vi "温度湿度监测界面.vi"() -> ()   [LabVIEW 2016, in "环境动力监测库.lvlib"]
uses:
  <vilib>/Utility/config.llb/NI_LVConfig.lvlib
  <vilib>/ptbypt/NI_PtbyPt.lvlib
panel:
  in  "解除告警":bool
  out "告警内容":string
  in  "高温告警启用":bool
  out "湿度显示":dbl=21.0 format="%.2f %%"
  out "湿度":dbl(graph)
  out "温度显示":dbl=21.0 format="%.2f ℃"
  out "温度":dbl(graph)
  in  "湿度下限告警点":dbl
  in  "湿度上限告警点":dbl
  in  "室温下限告警点":dbl
  in  "室温上限告警点":dbl
  # "℃"
  # "℃"
  # "%"
  # "%"
  # "温湿度监测"
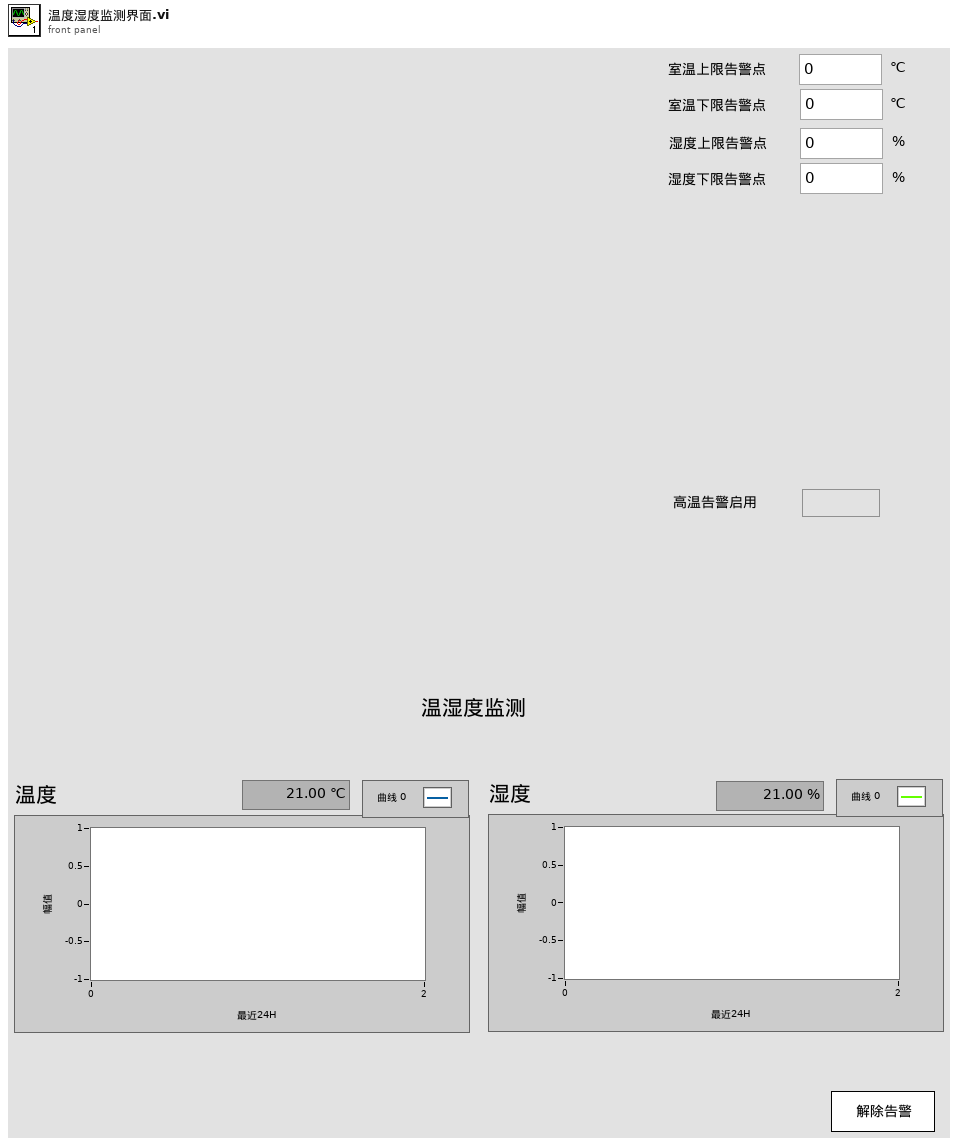
[diagram p1: front panel]
types:
  T1 = enum16{"报警状态监测", "报警确认", "仪器断电", "市电断电", "工控机关机", "取消告警", "结束"}
  T2 = typedef "NI_LVConfig.lvlib/Config Data RefNum.ctl" = refnum<k1>
  T3 = cluster{"漏水监测配置":cluster{"监测项描述:输出":string, "端口:":enum16{"AI0", "AI1", "AI2", "AI3", "AI4", "DI0", "DI1", "DI2", "DI3", "DI4", "DO0", "DO1", "DO2", "DO3", "DO4", "X0", "X1", "X2", "X3", "X4", "X5", "X6", "X7", "X8", "X9"}, "告警参数:":enum32{"禁用告警", "闭合告警", "断开告警"}, "传感器型号:":enum16{"PLC", "ZLAN"}, "声光告警启用":bool}, "门禁开关监测配置":cluster{"监测项描述:输出":string, "端口:":enum16{"AI0", "AI1", "AI2", "AI3", "AI4", "DI0", "DI1", "DI2", "DI3", "DI4", "DO0", "DO1", "DO2", "DO3", "DO4", "X0", "X1", "X2", "X3", "X4", "X5", "X6", "X7", "X8", "X9"}, "告警参数:":enum32{"禁用告警", "闭合告警", "断开告警"}, "传感器型号:":enum16{"PLC", "ZLAN"}, "声光告警启用":bool}, "门禁开关监测配置2":cluster{"监测项描述:输出":string, "端口:":enum16{"AI0", "AI1", "AI2", "AI3", "AI4", "DI0", "DI1", "DI2", "DI3", "DI4", "DO0", "DO1", "DO2", "DO3", "DO4", "X0", "X1", "X2", "X3", "X4", "X5", "X6", "X7", "X8", "X9"}, "告警参数:":enum32{"禁用告警", "闭合告警", "断开告警"}, "传感器型号:":enum16{"PLC", "ZLAN"}, "声光告警启用":bool}, "温湿度监测配置":cluster{"监测项描述:输出":string, "端口:":enum16{"AI0", "AI1", "AI2", "AI3", "AI4", "DI0", "DI1", "DI2", "DI3", "DI4", "DO0", "DO1", "DO2", "DO3", "DO4", "X0", "X1", "X2", "X3", "X4", "X5", "X6", "X7", "X8", "X9"}, "告警参数:":enum32{"禁用告警", "闭合告警", "断开告警"}, "传感器型号:":enum16{"PLC", "ZLAN"}, "声光告警启用":bool}, "烟雾监测配置":cluster{"监测项描述:输出":string, "端口:":enum16{"AI0", "AI1", "AI2", "AI3", "AI4", "DI0", "DI1", "DI2", "DI3", "DI4", "DO0", "DO1", "DO2", "DO3", "DO4", "X0", "X1", "X2", "X3", "X4", "X5", "X6", "X7", "X8", "X9"}, "告警参数:":enum32{"禁用告警", "闭合告警", "断开告警"}, "传感器型号:":enum16{"PLC", "ZLAN"}, "声光告警启用":bool}, "冰箱监测配置":cluster{"监测项描述:输出":string, "端口:":enum16{"AI0", "AI1", "AI2", "AI3", "AI4", "DI0", "DI1", "DI2", "DI3", "DI4", "DO0", "DO1", "DO2", "DO3", "DO4", "X0", "X1", "X2", "X3", "X4", "X5", "X6", "X7", "X8", "X9"}, "告警参数:":enum32{"禁用告警", "闭合告警", "断开告警"}, "传感器型号:":enum16{"PLC", "ZLAN"}, "声光告警启用":bool}, "排气扇监测配置":cluster{"监测项描述:输出":string, "端口:":enum16{"AI0", "AI1", "AI2", "AI3", "AI4", "DI0", "DI1", "DI2", "DI3", "DI4", "DO0", "DO1", "DO2", "DO3", "DO4", "X0", "X1", "X2", "X3", "X4", "X5", "X6", "X7", "X8", "X9"}, "告警参数:":enum32{"禁用告警", "闭合告警", "断开告警"}, "传感器型号:":enum16{"PLC", "ZLAN"}, "声光告警启用":bool}, "红外入侵监测配置":cluster{"监测项描述:输出":string, "端口:":enum16{"AI0", "AI1", "AI2", "AI3", "AI4", "DI0", "DI1", "DI2", "DI3", "DI4", "DO0", "DO1", "DO2", "DO3", "DO4", "X0", "X1", "X2", "X3", "X4", "X5", "X6", "X7", "X8", "X9"}, "告警参数:":enum32{"禁用告警", "闭合告警", "断开告警"}, "传感器型号:":enum16{"PLC", "ZLAN"}, "声光告警启用":bool}, "振动监测配置":cluster{"监测项描述:输出":string, "端口:":enum16{"AI0", "AI1", "AI2", "AI3", "AI4", "DI0", "DI1", "DI2", "DI3", "DI4", "DO0", "DO1", "DO2", "DO3", "DO4", "X0", "X1", "X2", "X3", "X4", "X5", "X6", "X7", "X8", "X9"}, "告警参数:":enum32{"禁用告警", "闭合告警", "断开告警"}, "传感器型号:":enum16{"PLC", "ZLAN"}, "声光告警启用":bool}}
  T4 = cluster{"监测项描述:输出":string, "端口:":enum16{"AI0", "AI1", "AI2", "AI3", "AI4", "DI0", "DI1", "DI2", "DI3", "DI4", "DO0", "DO1", "DO2", "DO3", "DO4", "X0", "X1", "X2", "X3", "X4", "X5", "X6", "X7", "X8", "X9"}, "告警参数:":enum32{"禁用告警", "闭合告警", "断开告警"}, "传感器型号:":enum16{"PLC", "ZLAN"}, "声光告警启用":bool}
  T5 = enum16{"AI0", "AI1", "AI2", "AI3", "AI4", "DI0", "DI1", "DI2", "DI3", "DI4", "DO0", "DO1", "DO2", "DO3", "DO4", "X0", "X1", "X2", "X3", "X4", "X5", "X6", "X7", "X8", "X9"}
  T6 = cluster{"状态":cluster{"R0":i16, "R1":i16, "R2":i16, "R3":i16, "R4":i16, "R5":i16, "R6":i16, "R7":i16, "R8":i16, "R9":i16, "R10":i16, "R11":i16, "R12":i16, "R13":i16, "R14":i16, "R15":i16, "R16":i16, "R17":i16, "R18":i16, "R19":i16, "R20":i16, "R21":i16, "R22":i16, "R23":i16, "R24":i16, "R25":i16, "R26":i16, "R27":i16, "R28":i16, "R29":i16, "R30":i16, "R31":i16, "R32":i16, "R33":i16, "R34":i16, "R35":i16, "R36":i16, "R37":i16, "R38":i16, "R39":i16}, "输入状态":bool[], "输出状态":bool[], "参数设置":cluster{"R100":i16, "R101":i16, "R102":i16, "R103":i16, "R104":i16, "R105":i16, "R106":i16, "R107":i16, "R108":i16, "R109":i16, "R110":i16, "R111":i16, "R112":i16, "R113":i16, "R114":i16, "R115":i16, "R116":i16, "R117":i16, "R118":i16, "R119":i16, "R120":i16, "R121":i16, "R122":i16, "R123":i16}, "转换值":cluster{"AD0":sgl, "AD1":sgl, "AD2":sgl, "AD3":sgl, "AD4":sgl, "AD5":sgl}}
  T7 = cluster{"状态":cluster{"R0":i16, "R1":i16, "R2":i16, "R3":i16, "R4":i16, "R5":i16, "R6":i16, "R7":i16, "R8":i16, "R9":i16, "R10":i16, "R11":i16, "R12":i16, "R13":i16, "R14":i16, "R15":i16, "R16":i16, "R17":i16, "R18":i16, "R19":i16, "R20":i16, "R21":i16, "R22":i16, "R23":i16, "R24":i16, "R25":i16, "R26":i16, "R27":i16, "R28":i16, "R29":i16, "R30":i16, "R31":i16, "R32":i16, "R33":i16, "R34":i16, "R35":i16, "R36":i16, "R37":i16, "R38":i16, "R39":i16, "R40":i16, "R41":i16, "R42":i16, "R43":i16, "R44":i16, "R45":i16, "R46":i16, "R47":i16, "R48":i16, "R49":i16, "R50":i16, "R51":i16, "R52":i16, "R53":i16, "R54":i16, "R55":i16, "R56":i16, "R57":i16, "R58":i16, "R59":i16, "R60":i16, "R61":i16, "R62":i16, "R63":i16, "R64":i16, "R65":i16, "R66":i16, "R67":i16, "R68":i16, "R69":i16}, "输入状态":bool[], "输出状态":bool[], "报警簇":bool[], "参数设置":cluster{"R100":i16, "R101":i16, "R102":i16, "R103":i16, "R104":i16, "R105":i16, "R106":i16, "R107":i16, "R108":i16, "R109":i16, "R110":i16, "R111":i16, "R112":i16, "R113":i16, "R114":i16, "R115":i16, "R116":i16, "R117":i16, "R118":i16, "R119":i16, "R120":i16, "R121":i16, "R122":i16, "R123":i16, "R124":i16}, "转换值":cluster{"AD0":sgl, "AD1":sgl, "AD2":sgl, "AD3":sgl, "AD4":sgl, "AD5":sgl}, "看门狗启用":bool, "氨氮模块名称":string, "总磷模块名称":string}
  T8 = cluster{"AD0":dbl, "AD1":dbl, "AD2":dbl, "AD3":dbl, "AD4":dbl, "AD5":dbl, "AD6":dbl, "AD7":dbl}
  T9 = cluster{"命令":string, cluster{"starting address":u16, "holding register value":u16}}
  T10 = cluster{"温湿度":cluster{"状态":bool, "温度:":sgl, "湿度:":sgl, "详情  ":bool}, "空调":cluster{"状态":bool, "机柜温度:":sgl, "压缩机:":enum16{"停止", "运行"}, "电加热:":enum16{"停止", "运行"}, "详情  ":bool}, "排气扇":cluster{"排气扇:":enum16{"关闭", "打开"}, "详情  ":bool}, "冰箱":cluster{"冰箱:":enum16{"关闭", "打开"}, "详情  ":bool}}
  T11 = cluster{"漏水监测输出":cluster{"漏水监测告警":bool, "告警内容":string}, "门禁监测输出":cluster{"门禁监测告警":bool, "告警内容":string}, "门禁监测输出2":cluster{"门禁监测告警":bool, "告警内容":string}, "温湿度监测输出":cluster{"温湿度监测告警":bool, "告警内容":string}, "烟雾监测输出":cluster{"烟雾监测告警":bool, "告警内容":string}, "空调监测输出":cluster{"空调监测告警":bool, "告警内容":string}, "自动重合闸输出":cluster{"自动重合闸告警":bool, "告警内容":string}, "红外入侵输出":cluster{"红外入侵告警":bool, "告警内容":string}, "振动输出":cluster{"振动告警":bool, "告警内容":string}, "UPS输出":cluster{"UPS告警":bool, "告警内容":string}, "蓄电池输出":cluster{"蓄电池告警":bool, "告警内容":string}, "蓄电池输出2":cluster{"蓄电池告警":bool, "告警内容":string}, "GPS输出":cluster{"定位告警":bool, "告警内容":string}, "北斗输出":cluster{"定位告警":bool, "告警内容":string}, "气象输出":cluster{"气象告警":bool, "告警内容":string}}
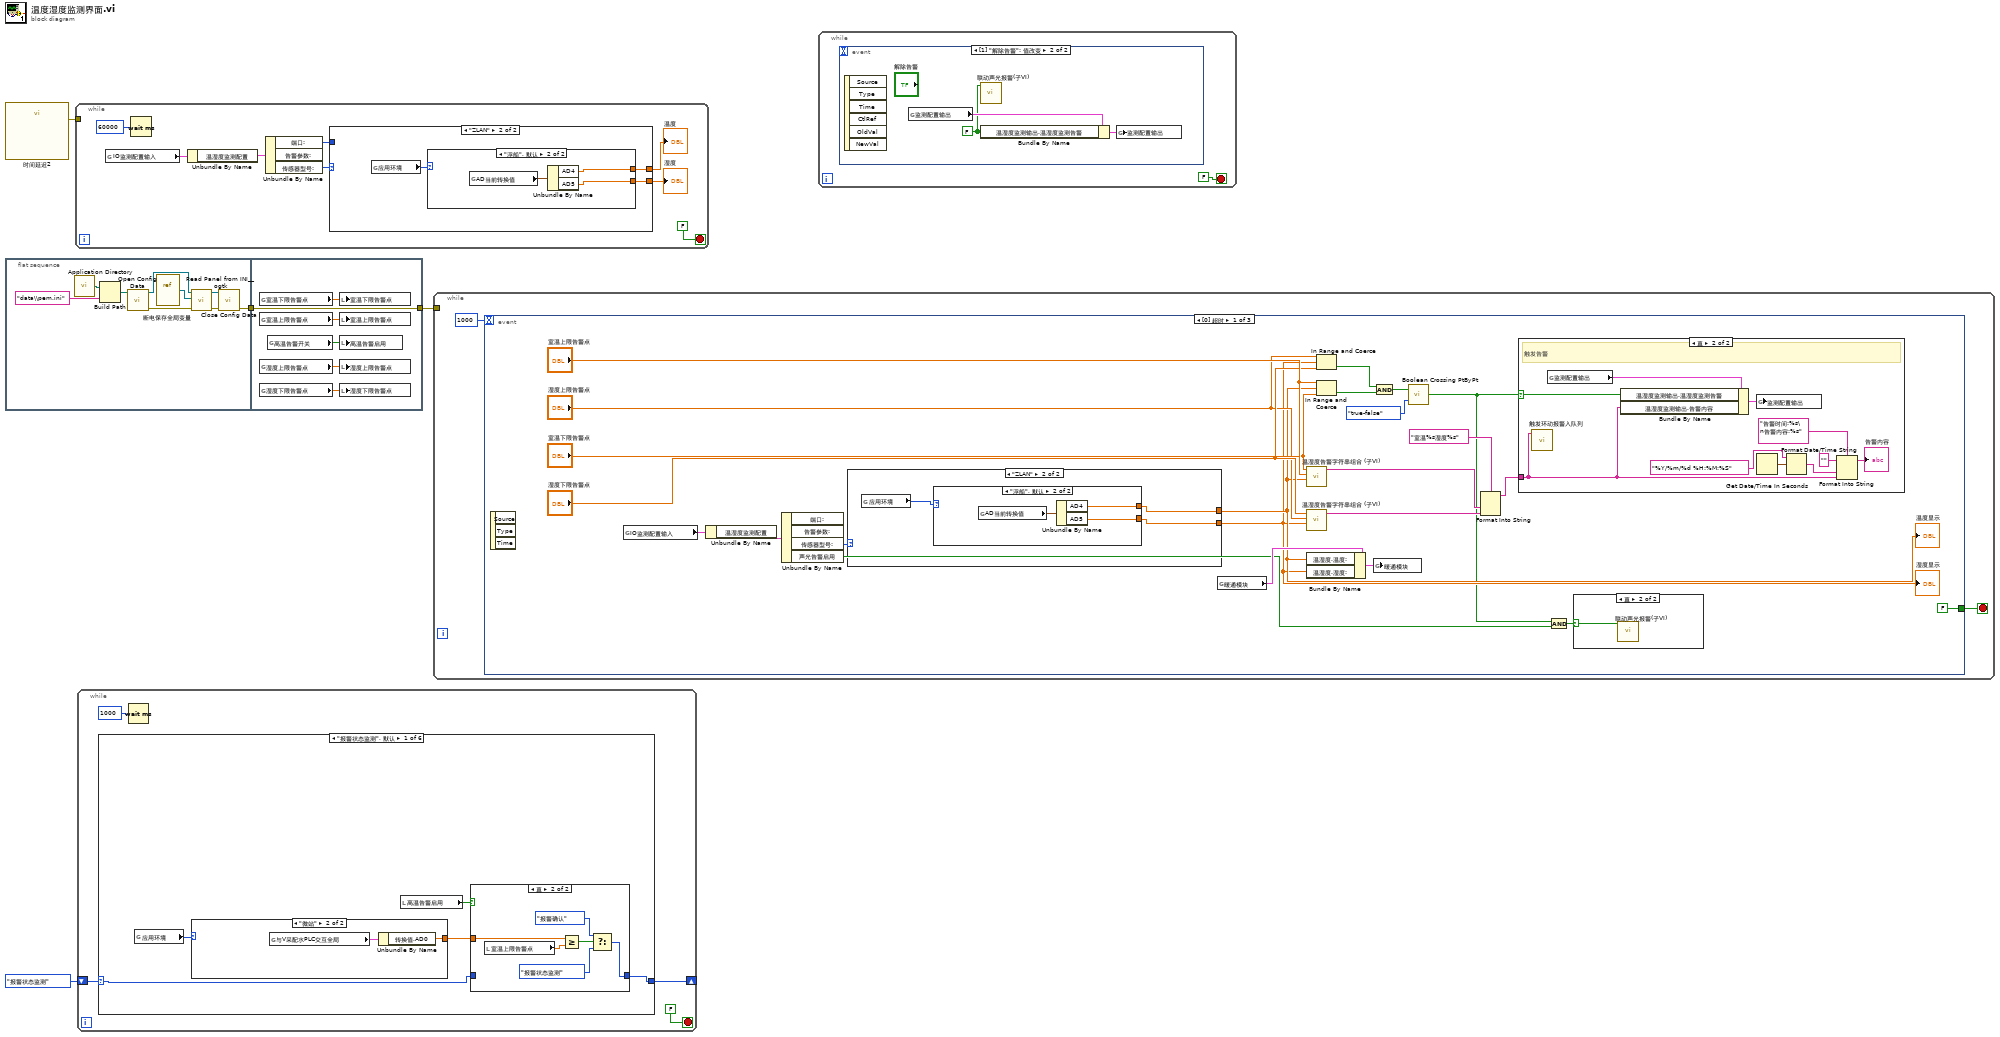
[diagram p0: block diagram]
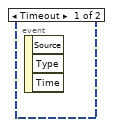
[diagram p2: hidden frame]
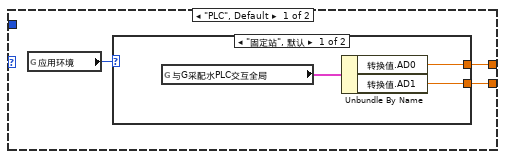
[diagram p3: hidden frame]
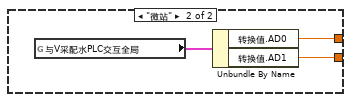
[diagram p4: hidden frame]
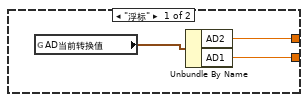
[diagram p5: hidden frame]
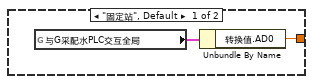
[diagram p6: hidden frame]
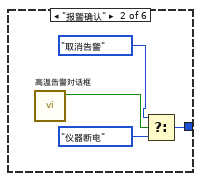
[diagram p8: hidden frame]
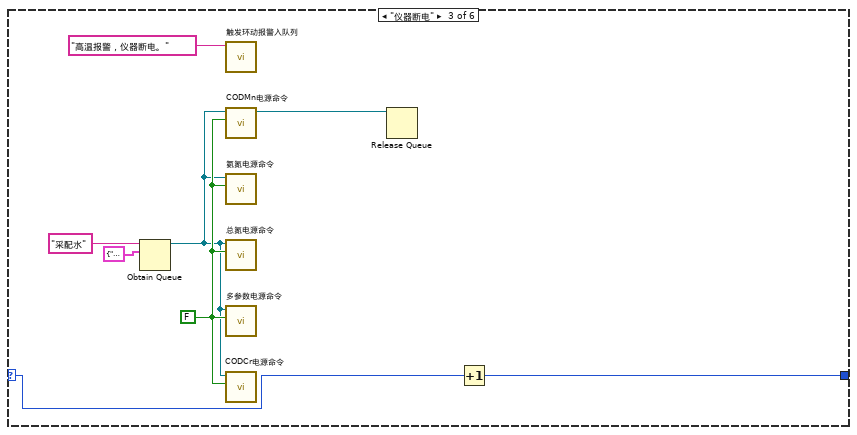
[diagram p9: hidden frame]
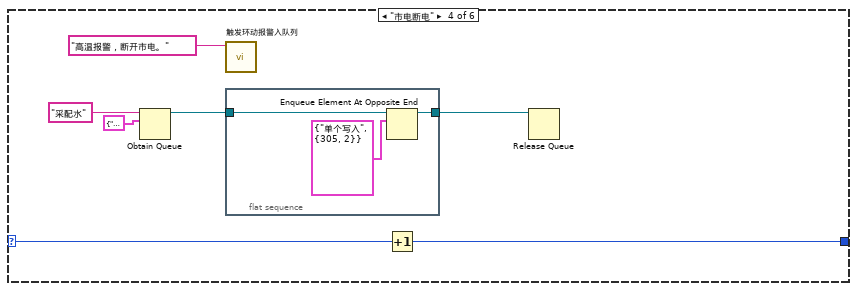
[diagram p10: hidden frame]
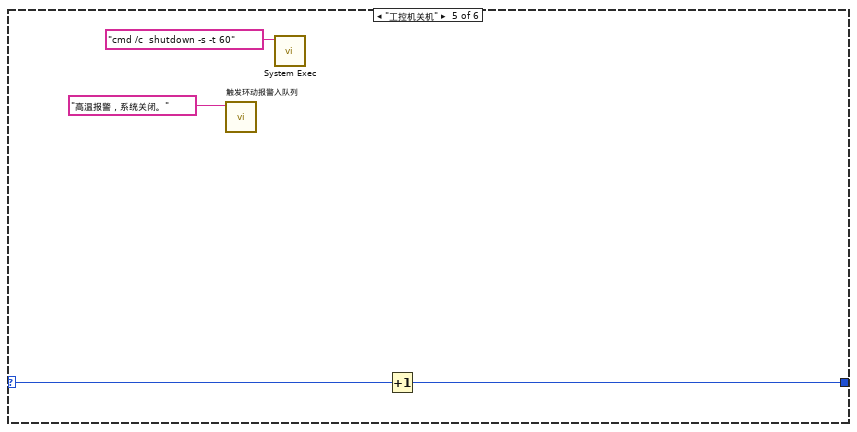
[diagram p11: hidden frame]
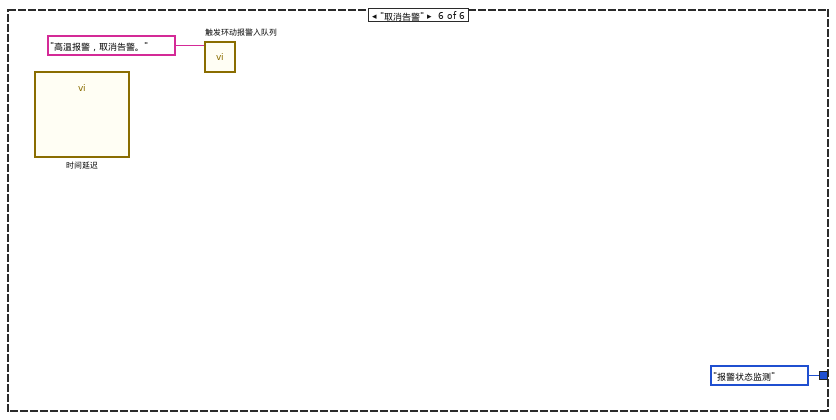
[diagram p12: hidden frame]
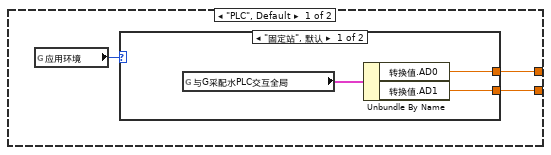
[diagram p14: hidden frame]
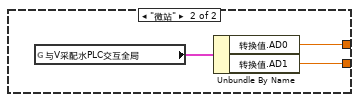
[diagram p15: hidden frame]
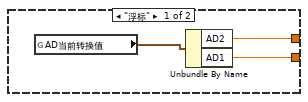
[diagram p16: hidden frame]
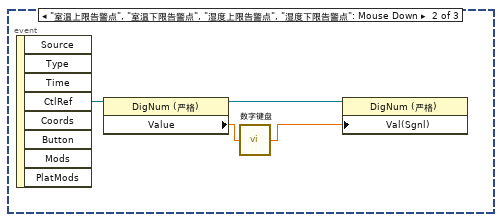
[diagram p18: hidden frame]
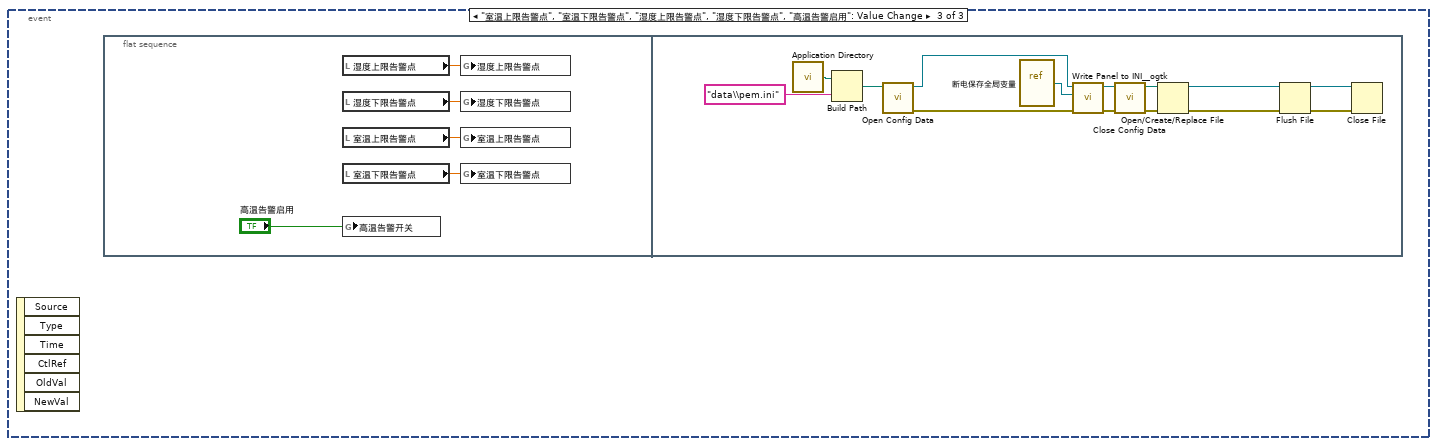
[diagram p19: hidden frame]
diagram:
  n1 = call "时间延迟2"() -> ("error out"=w1:errorcluster)  [unwired: 11 in]
  n2 = flat-sequence {
    tunnel: [w5] -> w4
    tunnel: [w19] -> w3
    tunnel: w4 -> [w19]
    frame #0 {
      n3 = call <vilib>:"Application Directory.vi"() -> ("Application Directory"=w13:path)
      n4 = Build Path(base path=w13, name or relative path="data\\pem.ini" ("名称或相对路径")) -> (appended path=w11:path)
      n5 = call <vilib>:"Open Config Data.vi"("configuration file path"=w11) -> ("error out"=w7:errorcluster, "refnum"=w10:T2)  [unwired: 8 in, 1 out]
      n6 = vi-ref "断电保存全局变量.vi"() -> (w9:refnum<vi>)
      n7 = call <userlib>:"Read Panel from INI__ogtk.vi"("error in (no error)"=w7, "VI ref"=w9, "refnum"=w10) -> ("error out"=w6:errorcluster, "refnum out"=w8:T2)  [unwired: 7 in]
      n8 = call <vilib>:"Close Config Data.vi"("error in (no error)"=w6, "refnum"=w8) -> ("error out"=w5:errorcluster)  [unwired: 8 in, 1 out]
    }
    frame #1 {
      n9 = global read "断电保存全局变量.vi" "室温下限告警点"() -> (w18:dbl)
      n10 = global read "断电保存全局变量.vi" "室温上限告警点"() -> (w17:dbl)
      n11 = global read "断电保存全局变量.vi" "湿度上限告警点"() -> (w15:dbl)
      n12 = global read "断电保存全局变量.vi" "湿度下限告警点"() -> (w16:dbl)
      n13 = global read "断电保存全局变量.vi" "高温告警开关"() -> (w14:bool)
      n14 = local write "室温下限告警点"(w18) -> ()
      n15 = local write "室温上限告警点"(w17) -> ()
      n16 = local write "高温告警启用"(w14) -> ()
      n17 = local write "湿度上限告警点"(w15) -> ()
      n18 = local write "湿度下限告警点"(w16) -> ()
    }
  }
  n19 = while {
    tunnel: w1 -> [_]
    stop <- FALSE stop-if-true
    n20 = global read "断电保存全局变量.vi" "IO监测配置输入"() -> (w20:T3)
    n21 = Wait (ms)(milliseconds to wait=u32 60000 ("等待时间（毫秒）")) -> ()  [unwired: 1 out]
    n22 = Unbundle By Name(w20) -> ("温湿度监测配置"=w25:T4)
    n23 = Unbundle By Name(w25) -> ("端口:"=w23:T5, "传感器型号:"=w24:enum16{"PLC", "ZLAN"})  [unwired: 1 out]
    n24 = case shown="\"ZLAN\"" w24 {
      tunnel: w23 -> [_ _]
      tunnel: [w29 w38] -> w22
      tunnel: [w28 w37] -> w21
      frame "PLC", Default {
        n25 = global read "外部交互全局变量.vi" "应用环境"() -> (w30:enum16{"固定站", "微站", "浮标", "浮船"})
        n26 = case shown="\"固定站\", 默认" w30 {
          tunnel: [w32 w35] -> w29
          tunnel: [w31 w34] -> w28
          frame "固定站", Default {
            n27 = global read "外部交互全局变量.vi" "与G采配水PLC交互全局"() -> (w33:T6)
            n28 = Unbundle By Name(w33) -> ("转换值.AD0"=w32:sgl, "转换值.AD1"=w31:sgl)
          }
          frame "微站" {
            n29 = global read "外部交互全局变量.vi" "与V采配水PLC交互全局"() -> (w36:T7)
            n30 = Unbundle By Name(w36) -> ("转换值.AD0"=w35:sgl, "转换值.AD1"=w34:sgl)
          }
        }
      }
      frame "ZLAN" {
        n31 = global read "外部交互全局变量.vi" "应用环境"() -> (w39:enum16{"固定站", "微站", "浮标", "浮船"})
        n32 = case shown="\"浮船\", 默认" w39 {
          tunnel: [w42 w44] -> w38
          tunnel: [w41 w43] -> w37
          frame "浮标" {
            n33 = global read "断电保存全局变量.vi" "AD当前转换值"() -> (w40:T8)
            n34 = Unbundle By Name(w40) -> ("AD2"=w42:dbl, "AD1"=w41:dbl)
          }
          frame "浮船", Default {
            n35 = global read "断电保存全局变量.vi" "AD当前转换值"() -> (w45:T8)
            n36 = Unbundle By Name(w45) -> ("AD4"=w44:dbl, "AD5"=w43:dbl)
          }
        }
      }
    }
    "温度" <- w22
    "湿度" <- w21
  }
  n37 = while {
    shift-right: [w49] -> _
    shift-left: T1."报警状态监测" ("枚举") -> [w48]
    stop <- FALSE stop-if-true
    n38 = case shown="\"报警状态监测\", 默认" w48 {
      selector: w48 -> [w52 _ w76 w79 w90 _]
      tunnel: [w54 w66 w75 w78 w89 T1."报警状态监测" ("枚举")] -> w49
      frame "报警状态监测", Default {
        n39 = global read "外部交互全局变量.vi" "应用环境"() -> (w51:enum16{"固定站", "微站", "浮标", "浮船"})
        n40 = case shown="\"微站\"" w51 {
          tunnel: [w55 w57] -> w50
          frame "固定站", Default {
            n41 = global read "外部交互全局变量.vi" "与G采配水PLC交互全局"() -> (w56:T6)
            n42 = Unbundle By Name(w56) -> ("转换值.AD0"=w55:sgl)
          }
          frame "微站" {
            n43 = global read "外部交互全局变量.vi" "与V采配水PLC交互全局"() -> (w58:T7)
            n44 = Unbundle By Name(w58) -> ("转换值.AD0"=w57:sgl)
          }
        }
        n45 = local read "高温告警启用"() -> (w53:bool)
        n46 = case shown="真" w53 {
          tunnel: [w59 w61] -> w54
          tunnel: w52 -> [w59 _]
          tunnel: w50 -> [_ w60]
          frame False {
          }
          frame True {
            n47 = local read "室温上限告警点"() -> (w65:dbl)
            n48 = Greater Or Equal?(x=w60, y=w65) -> (x >= y?=w64:bool)
            n49 = Select(t=T1."报警确认" ("枚举"), s=w64, f=T1."报警状态监测" ("枚举")) -> (s? t:f=w61:T1)
          }
        }
      }
      frame "报警确认" {
        n50 = call "高温告警对话框.vi"() -> ("T button?"=w67:bool)  [unwired: 11 in]
        n51 = Select(t=T1."取消告警" ("枚举"), s=w67, f=T1."仪器断电" ("枚举")) -> (s? t:f=w66:T1)
      }
      frame "仪器断电" {
        w74 = FALSE ("通电/断电")
        n52 = Obtain Queue(name (unnamed)="采配水" ("名称（未命名）"), element data type=cluster{"命令":string, "数据":variant} {"命令"="", "数据"=variant}) -> (queue out=w72:refnum<queue>)  [unwired: 3 in, 2 out]
        n53 = call "触发环动报警入队列.vi"("报警内容"="高温报警，仪器断电。" ("日志信息")) -> ()  [unwired: 11 in]
        n54 = call "CODMn电源命令.vi"("通电/断电"=w74, "队列"=w72) -> ("队列输出"=w73:refnum<queue>)  [unwired: 9 in]
        n55 = call "氨氮电源命令.vi"("通电/断电"=w74, "队列"=w72) -> ()  [unwired: 9 in, 1 out]
        n56 = call "总氮电源命令.vi"("通电/断电"=w74, "队列"=w72) -> ()  [unwired: 9 in, 1 out]
        n57 = call "多参数电源命令.vi"("通电/断电"=w74, "队列"=w72) -> ()  [unwired: 9 in, 1 out]
        n58 = call "CODCr电源命令.vi"("通电/断电"=w74, "队列"=w72) -> ()  [unwired: 9 in, 1 out]
        n59 = Release Queue(queue=w73) -> ()  [unwired: 2 in, 3 out]
        n60 = Increment(x=w76) -> (x+1=w75:T1)
      }
      frame "市电断电" {
        n61 = Obtain Queue(name (unnamed)="采配水" ("名称（未命名）"), element data type=cluster{"命令":string, "数据":variant} {"命令"="", "数据"=variant}) -> (queue out=w82:refnum<queue>)  [unwired: 3 in, 2 out]
        n62 = call "触发环动报警入队列.vi"("报警内容"="高温报警，断开市电。" ("日志信息")) -> ()  [unwired: 11 in]
        n63 = flat-sequence {
          tunnel: w82 -> [w86]
          tunnel: [w85] -> w81
          frame #0 {
            n64 = Enqueue Element At Opposite End(queue=w86, element=T9 {"命令"="单个写入", {"starting address"=305, "holding register value"=2}} ("元素")) -> (queue out=w85:refnum<queue>)  [unwired: 2 in, 2 out]
          }
        }
        n65 = Increment(x=w79) -> (x+1=w78:T1)
        n66 = Release Queue(queue=w81) -> ()  [unwired: 2 in, 3 out]
      }
      frame "工控机关机" {
        n67 = call "触发环动报警入队列.vi"("报警内容"="高温报警，系统关闭。" ("日志信息")) -> ()  [unwired: 11 in]
        n68 = call <vilib>:"System Exec.vi"("command line"="cmd /c  shutdown -s -t 60") -> ()  [unwired: 7 in, 4 out]
        n69 = Increment(x=w90) -> (x+1=w89:T1)
      }
      frame "取消告警" {
        n70 = call "时间延迟"() -> ()  [unwired: 11 in, 1 out]
        n71 = call "触发环动报警入队列.vi"("报警内容"="高温报警，取消告警。" ("日志信息")) -> ()  [unwired: 11 in]
      }
    }
    n72 = Wait (ms)(milliseconds to wait=u32 1000 ("等待时间（毫秒）")) -> ()  [unwired: 1 out]
  }
  n73 = while {
    tunnel: w3 -> [_]
    stop <- w95 stop-if-true
    n74 = event shown="[0] 超时" {
      selector: _ -> [_ _ _]
      dyn-events: _ -> [_ _ _]
      timeout: 1000 -> [_ _ _]
      tunnel: [FALSE _ _] -> w95
      event Timeout {
        n75 = event-data() -> ()  [unwired: 1 in, 3 out]
        n76 = global read "断电保存全局变量.vi" "IO监测配置输入"() -> (w105:T3)
        n77 = Unbundle By Name(w105) -> ("温湿度监测配置"=w116:T4)
        n78 = Unbundle By Name(w116) -> ("传感器型号:"=w104:enum16{"PLC", "ZLAN"}, "声光告警启用"=w96:bool)  [unwired: 2 out]
        n79 = case shown="\"ZLAN\"" w104 {
          tunnel: [w120 w130] -> w101
          tunnel: [w121 w129] -> w99
          frame "PLC", Default {
            n80 = global read "外部交互全局变量.vi" "应用环境"() -> (w122:enum16{"固定站", "微站", "浮标", "浮船"})
            n81 = case shown="\"固定站\", 默认" w122 {
              tunnel: [w124 w127] -> w120
              tunnel: [w123 w126] -> w121
              frame "固定站", Default {
                n82 = global read "外部交互全局变量.vi" "与G采配水PLC交互全局"() -> (w125:T6)
                n83 = Unbundle By Name(w125) -> ("转换值.AD0"=w124:sgl, "转换值.AD1"=w123:sgl)
              }
              frame "微站" {
                n84 = global read "外部交互全局变量.vi" "与V采配水PLC交互全局"() -> (w128:T7)
                n85 = Unbundle By Name(w128) -> ("转换值.AD0"=w127:sgl, "转换值.AD1"=w126:sgl)
              }
            }
          }
          frame "ZLAN" {
            n86 = global read "外部交互全局变量.vi" "应用环境"() -> (w131:enum16{"固定站", "微站", "浮标", "浮船"})
            n87 = case shown="\"浮船\", 默认" w131 {
              tunnel: [w134 w136] -> w130
              tunnel: [w133 w135] -> w129
              frame "浮标" {
                n88 = global read "断电保存全局变量.vi" "AD当前转换值"() -> (w132:T8)
                n89 = Unbundle By Name(w132) -> ("AD2"=w134:dbl, "AD1"=w133:dbl)
              }
              frame "浮船", Default {
                n90 = global read "断电保存全局变量.vi" "AD当前转换值"() -> (w137:T8)
                n91 = Unbundle By Name(w137) -> ("AD4"=w136:dbl, "AD5"=w135:dbl)
              }
            }
          }
        }
        "温度显示" <- w101
        "湿度显示" <- w99
        n92 = global read "内部交互全局变量.vi" "暖通模块"() -> (w103:T10)
        n93 = call "温湿度告警字符串组合 (子VI).vi"("AD01"=w101, "室温湿度上限告警点"="室温上限告警点", "室温湿度下限告警点"="室温下限告警点") -> ("字符串"=w108:string)  [unwired: 8 in]
        n94 = call "温湿度告警字符串组合 (子VI).vi"("AD01"=w99, "室温湿度上限告警点"="湿度上限告警点", "室温湿度下限告警点"="湿度下限告警点") -> ("字符串"=w107:string)  [unwired: 8 in]
        n95 = Bundle By Name(cluster=w103, "温湿度.温度:"=w101, "温湿度.湿度:"=w99) -> (w102:T10)
        n96 = In Range and Coerce(upper limit="湿度上限告警点", x=w99, lower limit="湿度下限告警点") -> (In Range?=w117:bool)  [unwired: 1 out]
        n97 = In Range and Coerce(upper limit="室温上限告警点", x=w101, lower limit="室温下限告警点") -> (In Range?=w114:bool)  [unwired: 1 out]
        n98 = global write "内部交互全局变量.vi" "暖通模块"(w102) -> ()
        n99 = And(x=w117, y=w114) -> (x .and. y?=w100:bool)
        n100 = call <vilib>:"Boolean Crossing PtByPt.vi"("direction"=enum16{"either", "false-true", "true-false"}."true-false", "input"=w100) -> ("crossing"=w97:bool)  [unwired: 1 in]
        n101 = Format Into String(format string="室温%s湿度%s" ("格式字符串"), w108, w107) -> (resulting string=w106:string)  [unwired: 2 in, 1 out]
        n102 = case shown="真" w97 {
          selector: w97 -> [_ w145]
          tunnel: w106 -> [_ w138]
          frame False {
          }
          frame True {
            # "触发告警"
            n103 = call "触发环动报警入队列.vi"("报警内容"=w138) -> ()  [unwired: 11 in]
            n104 = global read "断电保存全局变量.vi" "监测配置输出"() -> (w146:T11)
            n105 = Bundle By Name(cluster=w146, "温湿度监测输出.温湿度监测告警"=w145, "温湿度监测输出.告警内容"=w138) -> (w147:T11)
            n106 = global write "断电保存全局变量.vi" "监测配置输出"(w147) -> ()
            n107 = Get Date/Time In Seconds() -> (seconds since 1Jan1904=w141:timestamp)
            n108 = Format Date/Time String(time format string (%c)="%Y/%m/%d %H:%M:%S" ("时间格式字符串(%c)"), seconds (now)=w141) -> (date/time string=w143:string)  [unwired: 1 in]
            n109 = Format Into String(format string="告警时间:%s\n告警内容:%s" ("格式字符串"), initial string="" ("初始字符串"), w143, w138) -> (resulting string=→"告警内容":string)  [unwired: 1 in, 1 out]
          }
        }
        n110 = And(x=w97, y=w96) -> (x .and. y?=w98:bool)
        n111 = case shown="真" w98 {
          selector: w98 -> [_ w119]
          frame False {
          }
          frame True {
            n112 = call "联动声光报警(子VI).vi"("布尔"=w119) -> ()  [unwired: 11 in]
          }
        }
      }
      event "室温上限告警点", "室温下限告警点", "湿度上限告警点", "湿度下限告警点": Mouse Down {
        n113 = event-data() -> ("CtlRef"=w151:refnum<vi>)  [unwired: 1 in, 7 out]
        n114 = property class="DigNum (严格)"(reference=w151) -> (reference out=w149:refnum<vi>, "Value"=w150:dbl)  [unwired: 1 in, 1 out]
        n115 = call "数字键盘.vi"("OldNumber"=w150) -> ("NewNumber"=w148:sgl)
        n116 = property class="DigNum (严格)"(reference=w149, "Val(Sgnl)"=w148) -> ()  [unwired: 1 in, 2 out]
      }
      event "室温上限告警点", "室温下限告警点", "湿度上限告警点", "湿度下限告警点", "高温告警启用": Value Change {
        n117 = event-data() -> ()  [unwired: 1 in, 6 out]
        n118 = flat-sequence {
          frame #0 {
            n119 = local read "湿度上限告警点"() -> (w156:dbl)
            n120 = local read "湿度下限告警点"() -> (w155:dbl)
            n121 = local read "室温上限告警点"() -> (w154:dbl)
            n122 = local read "室温下限告警点"() -> (w153:dbl)
            n123 = global write "断电保存全局变量.vi" "高温告警开关"("高温告警启用") -> ()
            n124 = global write "断电保存全局变量.vi" "湿度上限告警点"(w156) -> ()
            n125 = global write "断电保存全局变量.vi" "湿度下限告警点"(w155) -> ()
            n126 = global write "断电保存全局变量.vi" "室温上限告警点"(w154) -> ()
            n127 = global write "断电保存全局变量.vi" "室温下限告警点"(w153) -> ()
          }
          frame #1 {
            n128 = call <vilib>:"Application Directory.vi"() -> ("Application Directory"=w169:path)
            n129 = Build Path(base path=w169, name or relative path="data\\pem.ini" ("名称或相对路径")) -> (appended path=w168:path)
            n130 = call <vilib>:"Open Config Data.vi"("configuration file path"=w168) -> ("error out"=w164:errorcluster, "refnum"=w167:T2)  [unwired: 8 in, 1 out]
            n131 = vi-ref "断电保存全局变量.vi"() -> (w166:refnum<vi>)
            n132 = call <userlib>:"Write Panel to INI__ogtk.vi"("error in (no error)"=w164, "VI ref"=w166, "refnum"=w167) -> ("error out"=w163:errorcluster, "refnum out"=w165:T2)  [unwired: 7 in]
            n133 = call <vilib>:"Close Config Data.vi"("error in (no error)"=w163, "refnum"=w165) -> ("error out"=w158:errorcluster, "file path"=w157:path)  [unwired: 8 in]
            n134 = Open/Create/Replace File(file path (use dialog)=w157, error in=w158) -> (refnum out=w161:refnum<file>, error out=w162:errorcluster)  [unwired: 4 in, 1 out]
            n135 = Flush File(refnum=w161, error in=w162) -> (refnum out=w160:refnum<file>, error out=w159:errorcluster)
            n136 = Close File(refnum=w160, error in=w159) -> ()  [unwired: 2 out]
          }
        }
      }
    }
  }
  n137 = while {
    stop <- FALSE stop-if-true
    n138 = event shown="[1] \"解除告警\": 值改变" {
      selector: _ -> [_ _]
      dyn-events: _ -> [_ _]
      timeout: _ -> [_ _]
      event Timeout {
        n139 = event-data() -> ()  [unwired: 1 in, 3 out]
      }
      event "解除告警": Value Change {
        w172 = FALSE
        n140 = event-data() -> ()  [unwired: 1 in, 6 out]
        n141 = global read "断电保存全局变量.vi" "监测配置输出"() -> (w173:T11)
        n142 = call "联动声光报警(子VI).vi"("布尔"=w172) -> ()  [unwired: 11 in]
        n143 = Bundle By Name(cluster=w173, "温湿度监测输出.温湿度监测告警"=w172) -> (w174:T11)
        n144 = global write "断电保存全局变量.vi" "监测配置输出"(w174) -> ()
      }
    }
  }
